vi "Get IO Names.vi"() -> (0 "AO Names":string[](array[string]), 1 "AI Names":string[](array[string]), 2 "DO Names":string[](array[string]), 3 "DI Names":string[](array[string]))   [LabVIEW 2014]
uses:
  Digital/Digital Input Cluster.ctl
  Digital/Digital Output Cluster.ctl
  Analog/Analog Output Cluster.ctl
  Analog/Analog Input Cluster.ctl
  Analog/Analog Result Cluster.ctl
panel:
  out "NI Analog Input":T1 {"Analog Result"."Számolt NTC hõmérséklet" format="%.3g"; "Analog Result"."15V" format="%.3g"; "Analog Result"."Elvárt NTC ellenállás" format="%.3g"; "Analog Result"."48V" format="%.3g"; "Analog Result"."Hõmérséklet" format="%.3g"; "Analog Result"."Szigetelési ellenállás" format="%.3g"; "Analog Result"."NTC ellenállás" format="%.3g"; "Analog Result"."Szenzor ellenállás" format="%.3g"}
  in  "NI Analog Output":T3
  out "concatenated string 3":string
  out "concatenated string 4":string
  out "concatenated string 2":string
  out "concatenated string":string
  in  "Digital Out":T4
  out "Digital input":T5
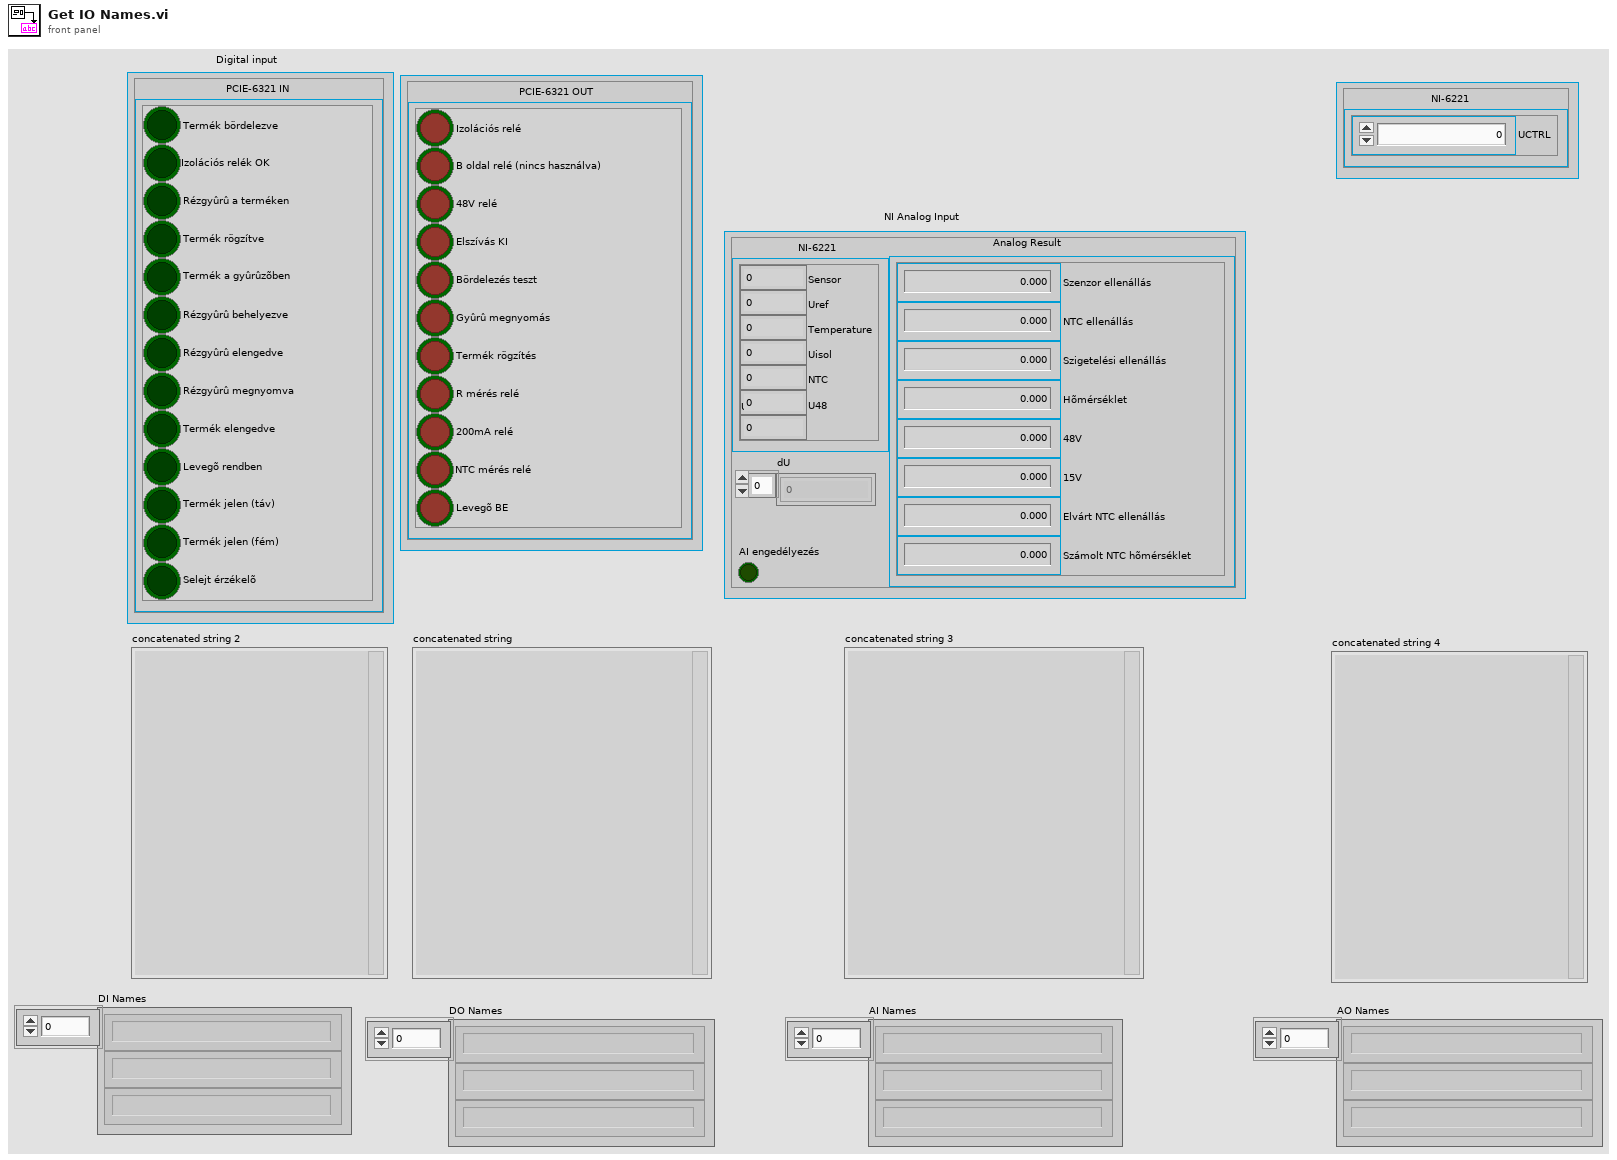
[diagram p1: front panel]
types:
  T1 = typedef "Analog Input Cluster.ctl" = cluster{"NI-6221":cluster{"Sensor":dbl, "Uref":dbl, "Temperature":dbl, "Uisol":dbl, "NTC":dbl, "U48":dbl, "U15":dbl}, "Analog Result":T2, "AI engedélyezés":bool, "dU":dbl[]}
  T2 = typedef "Analog Result Cluster.ctl" = cluster{"Szenzor ellenállás":dbl, "NTC ellenállás":dbl, "Szigetelési ellenállás":dbl, "Hõmérséklet":dbl, "48V":dbl, "15V":dbl, "Elvárt NTC ellenállás":dbl, "Számolt NTC hõmérséklet":dbl}
  T3 = typedef "Analog Output Cluster.ctl" = cluster{"NI-6221":cluster{"UCTRL":dbl}}
  T4 = typedef "Digital Output Cluster.ctl" = cluster{"PCIE-6321 OUT":cluster{"Izolációs relé":bool, "B oldal relé (nincs használva)":bool, "48V relé":bool, "Elszívás KI":bool, "Bördelezés teszt":bool, "Gyûrû megnyomás":bool, "Termék rögzítés":bool, "R mérés relé":bool, "200mA relé":bool, "NTC mérés relé":bool, "Levegõ BE":bool}}
  T5 = typedef "Digital Input Cluster.ctl" = cluster{"PCIE-6321 IN":cluster{"Termék bördelezve":bool, "Izolációs relék OK":bool, "Rézgyûrû a terméken":bool, "Termék rögzítve":bool, "Termék a gyûrûzõben":bool, "Rézgyûrû behelyezve":bool, "Rézgyûrû elengedve":bool, "Rézgyûrû megnyomva":bool, "Termék elengedve":bool, "Levegõ rendben":bool, "Termék jelen (táv)":bool, "Termék jelen (fém)":bool, "Selejt érzékelõ":bool}}
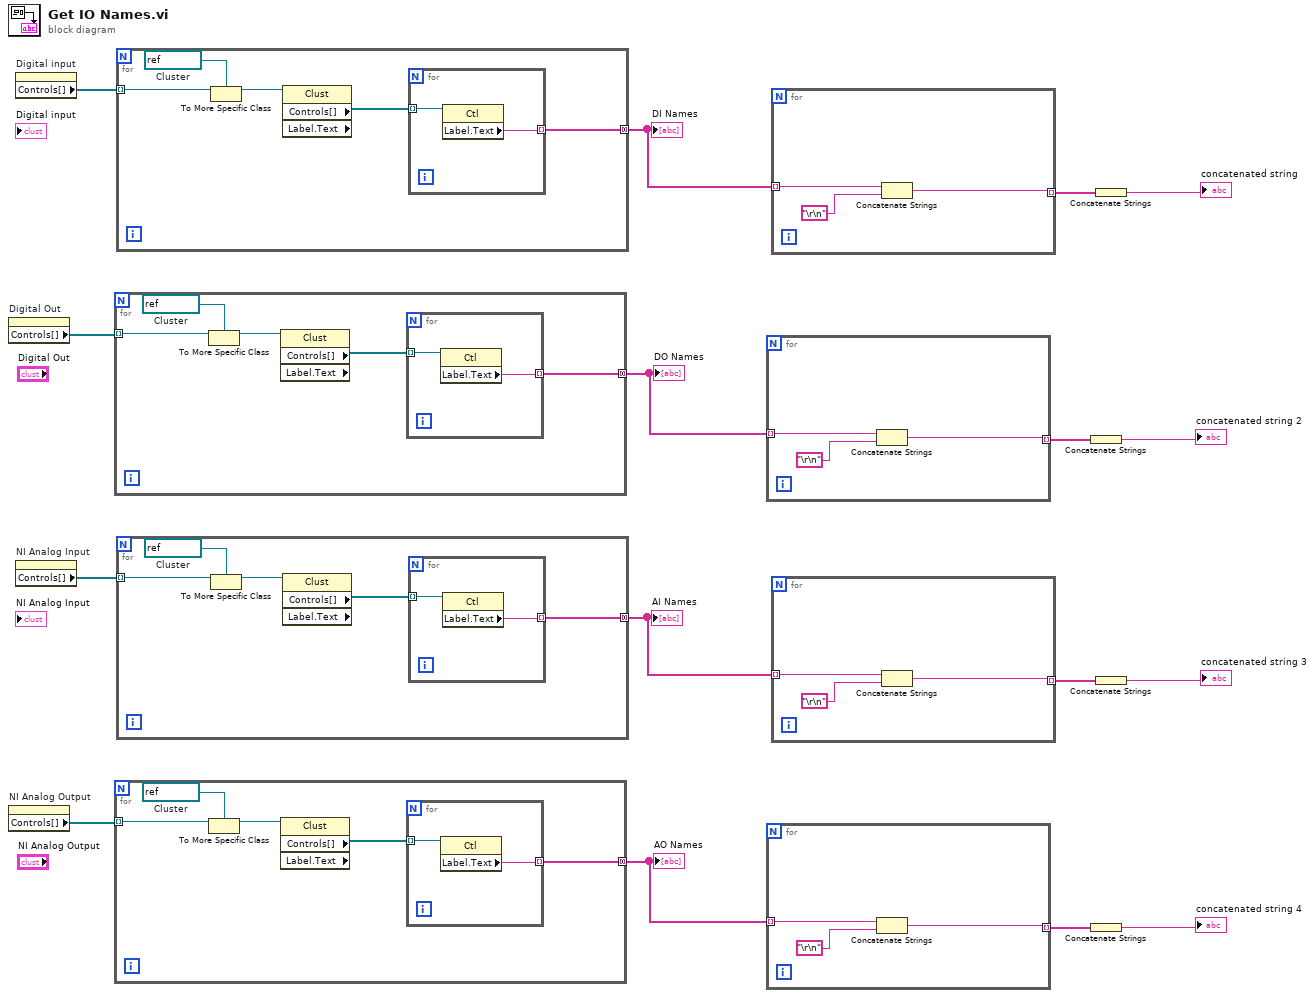
[diagram p0: block diagram]
diagram:
  n1 = property on="Digital Out" class="Clust (strict)"() -> ("Controls[]"=w12:refnum<vi>[])  [unwired: 2 in, 2 out]
  n2 = property on="NI Analog Output" class="Clust (strict)"() -> ("Controls[]"=w5:refnum<vi>[])  [unwired: 2 in, 2 out]
  n3 = property on="Digital input" class="Clust (strict)"() -> ("Controls[]"=w16:refnum<vi>[])  [unwired: 2 in, 2 out]
  n4 = property on="NI Analog Input" class="Clust (strict)"() -> ("Controls[]"=w1:refnum<vi>[])  [unwired: 2 in, 2 out]
  n5 = for {
    tunnel: w12 -> [w18] mode=indexing
    tunnel: [w17] -> w9 mode=concatenating
    w21 = refnum<vi> refnum  # Cluster
    n6 = To More Specific Class(target class=w21, reference=w18) -> (specific class reference=w20:refnum<vi>)  [unwired: 1 in, 1 out]
    n7 = property class="Clust" props=["Controls[]", "Label", "Text"](reference=w20) -> ("Controls[]"=w19:refnum<vi>[])  [unwired: 1 in, 3 out]
    n8 = for {
      tunnel: w19 -> [w23] mode=indexing
      tunnel: [w22] -> w17 mode=indexing
      n9 = property class="Ctl"(reference=w23) -> ("Label.Text"=w22:string)  [unwired: 1 in, 2 out]
    }
  }
  "DO Names" <- w9
  n10 = for {
    tunnel: w5 -> [w25] mode=indexing
    tunnel: [w24] -> w8 mode=concatenating
    w28 = refnum<vi> refnum  # Cluster
    n11 = To More Specific Class(target class=w28, reference=w25) -> (specific class reference=w27:refnum<vi>)  [unwired: 1 in, 1 out]
    n12 = property class="Clust" props=["Controls[]", "Label", "Text"](reference=w27) -> ("Controls[]"=w26:refnum<vi>[])  [unwired: 1 in, 3 out]
    n13 = for {
      tunnel: w26 -> [w30] mode=indexing
      tunnel: [w29] -> w24 mode=indexing
      n14 = property class="Ctl"(reference=w30) -> ("Label.Text"=w29:string)  [unwired: 1 in, 2 out]
    }
  }
  "AO Names" <- w8
  n15 = for {
    tunnel: w16 -> [w32] mode=indexing
    tunnel: [w31] -> w15 mode=concatenating
    w35 = refnum<vi> refnum  # Cluster
    n16 = To More Specific Class(target class=w35, reference=w32) -> (specific class reference=w34:refnum<vi>)  [unwired: 1 in, 1 out]
    n17 = property class="Clust" props=["Controls[]", "Label", "Text"](reference=w34) -> ("Controls[]"=w33:refnum<vi>[])  [unwired: 1 in, 3 out]
    n18 = for {
      tunnel: w33 -> [w37] mode=indexing
      tunnel: [w36] -> w31 mode=indexing
      n19 = property class="Ctl"(reference=w37) -> ("Label.Text"=w36:string)  [unwired: 1 in, 2 out]
    }
  }
  "DI Names" <- w15
  n20 = for {
    tunnel: w1 -> [w39] mode=indexing
    tunnel: [w38] -> w2 mode=concatenating
    w42 = refnum<vi> refnum  # Cluster
    n21 = To More Specific Class(target class=w42, reference=w39) -> (specific class reference=w41:refnum<vi>)  [unwired: 1 in, 1 out]
    n22 = property class="Clust" props=["Controls[]", "Label", "Text"](reference=w41) -> ("Controls[]"=w40:refnum<vi>[])  [unwired: 1 in, 3 out]
    n23 = for {
      tunnel: w40 -> [w44] mode=indexing
      tunnel: [w43] -> w38 mode=indexing
      n24 = property class="Ctl"(reference=w44) -> ("Label.Text"=w43:string)  [unwired: 1 in, 2 out]
    }
  }
  "AI Names" <- w2
  n25 = for {
    tunnel: w9 -> [w47] mode=indexing
    tunnel: [w45] -> w10 mode=indexing
    n26 = Concatenate Strings(w47, "\r\n") -> (w45:string)
  }
  n27 = for {
    tunnel: w8 -> [w50] mode=indexing
    tunnel: [w48] -> w7 mode=indexing
    n28 = Concatenate Strings(w50, "\r\n") -> (w48:string)
  }
  n29 = for {
    tunnel: w15 -> [w53] mode=indexing
    tunnel: [w51] -> w14 mode=indexing
    n30 = Concatenate Strings(w53, "\r\n") -> (w51:string)
  }
  n31 = for {
    tunnel: w2 -> [w56] mode=indexing
    tunnel: [w54] -> w3 mode=indexing
    n32 = Concatenate Strings(w56, "\r\n") -> (w54:string)
  }
  n33 = Concatenate Strings(w10) -> (→"concatenated string 2":string)
  n34 = Concatenate Strings(w7) -> (→"concatenated string 4":string)
  n35 = Concatenate Strings(w14) -> (→"concatenated string":string)
  n36 = Concatenate Strings(w3) -> (→"concatenated string 3":string)
